vi "SimpleDemo - backup.vi"() -> ()   [LabVIEW 2011]
uses:
  C:/Users/Behavior Room/Desktop/Kinect Mouse/DepthSense/FunctionPointerProxy/FunctionPointerProxy/obj/Release/FunctionPointerProxy.dll
  FunctionPointerProxy/FunctionPointerProxy/obj/Release/FunctionPointerProxy.dll
  <userlib>/libOptrima-2-3/libOptrima-2-3.lvlib
  <vilib>/vision/Image Controls.llb/IMAQ Image.ctl
  Program Files (x86)/SoftKinetic/OptrimaSDK/lib/libOptrima-2-3.dll
  <vilib>/Platform/TimedLoop/XDataNode/XDataNode.xnode
  <vilib>/Platform/TimedLoop/XDataNode/nitl_modes.ctl
  <vilib>/Platform/TimedLoop/XDataNode/XDNodeRunTimeDep.lvlib
  <vilib>/Platform/TimedLoop/XDataNode/wakeup.ctl
  <vilib>/Platform/TimedLoop/XDataNode/timing_clust.ctl
panel:
  out "API version":string
  out "array length":i32
  out "Image":T1(plugin-control)
  out "add newframe\ncallback":i32
  in  "stop":bool
  in  "Buffer Size 3":i32=10
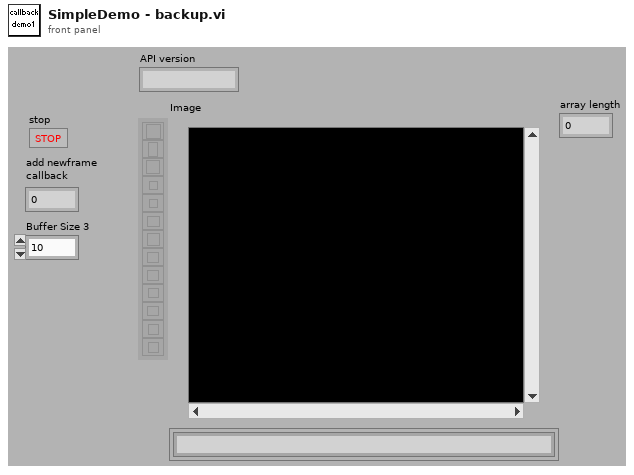
[diagram p1: front panel]
types:
  T1 = typedef "IMAQ Image.ctl" = refnum<image>
  T2 = typedef "XDNodeRunTimeDep.lvlib/timing_clust.ctl" = cluster{"Expected End [f-1]":u64, "Actual End [f-1]":u64, "Finished Late? [f-1]":bool, "Expected End [i-1]":u64, "Actual End [i-1]":u64, "Finished Late? [i-1]":bool, "Expected Start [i]":u64, "Actual Start [i]":u64, "Expected Start [f]":u64, "Actual Start [f]":u64, "Source Name":string, "Structure Name":string, "Period":i64, "Deadline":i64, "Offset":i64, "Start":i64, "Priority":i32, "Timeout":i32, "Mode":T3, "Wakeup Reason":T4, "Error":errorcluster, "Source Type":string, "Secondary Source Type":string, "Global End Time":u64, "Global Start Time":u64, "Frame Duration":u64, "Iteration Duration":u64, "Assigned CPU":i32, "I/O Scan Engine Mode":u32}
  T3 = typedef "XDNodeRunTimeDep.lvlib/nitl_modes.ctl" = enum32{"No Change", "Process missed periods, maintain original phase", "Discard missed periods, maintain original phase", "Process missed periods, ignore original phase", "Discard missed periods, ignore original phase"}
  T4 = typedef "XDNodeRunTimeDep.lvlib/wakeup.ctl" = enum32{"Normal", "Aborted", "Asynchronous wakeup", "Timing source error", "Timed loop error", "Timeout"}
  T5 = cluster{"queue out":refnum<queue>, "queue out":refnum<queue>}
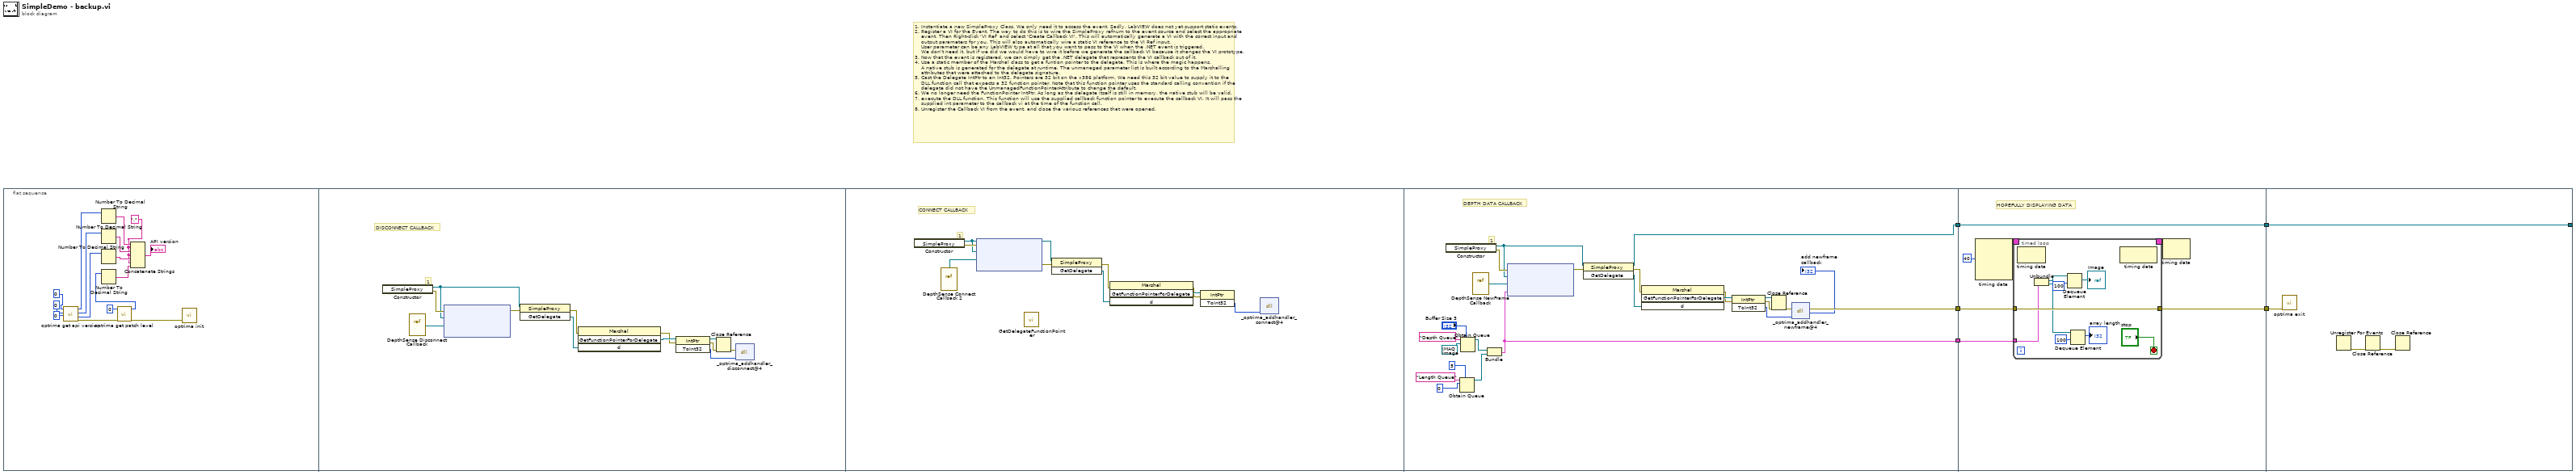
[diagram p0: block diagram]
diagram:
  # "1. Instantiate a new SimpleProxy Class. We only need it to access the event. Sadly, LabVIEW does not yet support static events.\n2. Register a VI for the Event. The way to do this is to wire the SimpleProxy refnum to the event source and select the appropriate\n    event. Then Right-click 'VI Ref' and select 'Create Callback VI'. This will automatically generate a VI with the correct input and\n    output parameters for you. This will also automatically wire a static VI reference to the VI Ref input.\n    User parameter can be any LabVIEW type at all that you want to pass to the VI when the .NET event is triggered.\n    We don't need it, but if we did we would have to wire it before we generate the callback VI because it changes the VI prototype.\n3. Now that the event is registered, we can simply get the .NET delegate that represents the VI callback out of it.\n4. Use a static member of the Marshal class to get a funtion pointer to the delegate. This is where the magic happens.\n    A native stub is generated for the delegate at runtime. The unmanaged parameter list is built according to the Marshalling\n    attributes that were attached to the delegate signature.\n5. Cast the Delegate IntPtr to an Int32. Pointers are 32 bit on the x386 platform. We need this 32 bit value to supply it to the\n    DLL function call that expects a 32 function pointer. Note that this function pointer uses the standard calling convention if the\n    delegate did not have the UnmanagedFunctionPointerAttribute to change the default.\n6. We no longer need the FunctionPointer IntPtr. As long as the delegate itself is still in memory, the native stub will be valid.\n7. execute the DLL function. This function will use the supplied callback function pointer to execute the callback VI. It will pass the\n    supplied int parameter to the callback vi at the time of the function call.\n8. Unregister the Callback VI from the event, and close the various references that were opened."
  n1 = flat-sequence {
    tunnel: [w66] -> w5
    tunnel: [w64] -> w4
    tunnel: [w44] -> w3
    tunnel: w5 -> [w73]
    tunnel: w4 -> [w71]
    tunnel: w3 -> [w70]
    tunnel: [w72] -> w2
    tunnel: [w71] -> w1
    tunnel: [w92] -> _
    tunnel: w2 -> [w91]
    tunnel: w1 -> [w92]
    frame #0 {
      w6 = "."
      n2 = call <userlib>:"optrima get api version.vi"("minor"=u32 0, "major"=u32 0, "release"=u32 0) -> ("error out"=w21:errorcluster, "minor out"=w17:u32, "major out"=w18:u32, "release out"=w19:u32)  [unwired: 5 in]
      n3 = Number To Decimal String(number=w19) -> (decimal integer string=w15:string)  [unwired: 1 in]
      n4 = Number To Decimal String(number=w18) -> (decimal integer string=w9:string)  [unwired: 1 in]
      n5 = Number To Decimal String(number=w17) -> (decimal integer string=w8:string)  [unwired: 1 in]
      n6 = call <userlib>:"optrima get patch level.vi"("error in (no error)"=w21, "patch"=u32 0) -> ("error out"=w20:errorcluster, "patch out"=w16:u32)  [unwired: 8 in]
      n7 = Number To Decimal String(number=w16) -> (decimal integer string=w7:string)  [unwired: 1 in]
      n8 = Concatenate Strings(w15, w6, w9, w6, w8, w6, w7) -> (→"API version":string)
      n9 = call <userlib>:"optrima init.vi"("error in (no error)"=w20) -> ()  [unwired: 10 in, 1 out]
    }
    frame #1 {
      # "DISCONNECT CALLBACK"
      # "1"
      n10 = constructor class="SimpleProxy"() -> (reference out=w25:refnum<k24>, error out=w29:errorcluster)  [unwired: 3 in, 1 out]
      n11 = vi-ref "DepthSense Disconnect Callback.vi"() -> ("vi reference"=w23:refnum<vi>)
      n12 = node(w29, w25, w23) -> (w33:errorcluster)  [unwired: 2 in, 1 out]
      n13 = invoke class="SimpleProxy" method="GetDelegate"(reference=w25, error in=w33) -> (error out=w31:errorcluster, "GetDelegate"=w22:refnum<k24>)  [unwired: 1 in, 1 out]
      n14 = invoke class="Marshal" method="GetFunctionPointerForDelegate"(error in=w31, "d"=w22) -> (error out=w30:errorcluster, "GetFunctionPointerForDelegate"=w32:refnum<k24>)  [unwired: 2 in, 2 out]
      n15 = invoke class="IntPtr" method="ToInt32"(reference=w32, error in=w30) -> (reference out=w28:refnum<k24>, error out=w26:errorcluster, "ToInt32"=w24:i32)  [unwired: 1 in]
      n16 = Close Reference(reference=w28, error in (no error)=w26) -> (error out=w27:errorcluster)
      n17 = dll-call lib="C:/Program Files (x86)/SoftKinetic/OptrimaSDK/lib/libOptrima-2-3.dll" fn="_optrima_addhandler_disconnect@4"(error in=w27, "handlerfunc"=w24) -> ()  [unwired: 4 in, 2 out]
    }
    frame #2 {
      # "CONNECT CALLBACK"
      # "1"
      n18 = constructor class="SimpleProxy"() -> (reference out=w37:refnum<k24>, error out=w38:errorcluster)  [unwired: 3 in, 1 out]
      n19 = vi-ref "DepthSense Connect Callback 2.vi"() -> ("vi reference"=w35:refnum<vi>)
      n20 = node(w38, w37, w35) -> (w42:errorcluster)  [unwired: 2 in, 1 out]
      n21 = call "GetDelegateFunctionPointer.vi"() -> ()  [unwired: 9 in, 3 out]
      n22 = invoke class="SimpleProxy" method="GetDelegate"(reference=w37, error in=w42) -> (error out=w40:errorcluster, "GetDelegate"=w34:refnum<k24>)  [unwired: 1 in, 1 out]
      n23 = invoke class="Marshal" method="GetFunctionPointerForDelegate"(error in=w40, "d"=w34) -> (error out=w39:errorcluster, "GetFunctionPointerForDelegate"=w41:refnum<k24>)  [unwired: 2 in, 2 out]
      n24 = invoke class="IntPtr" method="ToInt32"(reference=w41, error in=w39) -> ("ToInt32"=w36:i32)  [unwired: 1 in, 2 out]
      n25 = dll-call lib="C:/Program Files (x86)/SoftKinetic/OptrimaSDK/lib/libOptrima-2-3.dll" fn="_optrima_addhandler_connect@4"("handlerfunc"=w36) -> ()  [unwired: 5 in, 2 out]
    }
    frame #3 {
      # "DEPTH DATA CALLBACK"
      # "1"
      n26 = constructor class="SimpleProxy"() -> (reference out=w55:refnum<k24>, error out=w59:errorcluster)  [unwired: 3 in, 1 out]
      n27 = Obtain Queue(max queue size (-1, unlimited)=5, name (unnamed)="Length Queue", element data type=0) -> (queue out=w45:refnum<queue>)  [unwired: 2 in, 2 out]
      n28 = Obtain Queue(max queue size (-1, unlimited)="Buffer Size 3", name (unnamed)="Depth Queue", element data type=T1 refnum ("New Image")) -> (queue out=w49:refnum<queue>)  [unwired: 2 in, 2 out]
      n29 = vi-ref "DepthSense NewFrame Callback.vi"() -> ("vi reference"=w43:refnum<vi>)
      n30 = Bundle("queue out"=w49, "queue out"=w45) -> (w44:T5)  [unwired: 1 in]
      n31 = node(w59, w55, w43, w44) -> (w63:errorcluster)  [unwired: 1 in, 1 out]
      n32 = invoke class="SimpleProxy" method="GetDelegate"(reference=w55, error in=w63) -> (reference out=w64:refnum<k24>, error out=w61:errorcluster, "GetDelegate"=w65:refnum<k24>)  [unwired: 1 in]
      n33 = invoke class="Marshal" method="GetFunctionPointerForDelegate"(error in=w61, "d"=w65) -> (error out=w60:errorcluster, "GetFunctionPointerForDelegate"=w62:refnum<k24>)  [unwired: 2 in, 2 out]
      n34 = invoke class="IntPtr" method="ToInt32"(reference=w62, error in=w60) -> (reference out=w58:refnum<k24>, error out=w56:errorcluster, "ToInt32"=w54:i32)  [unwired: 1 in]
      n35 = Close Reference(reference=w58, error in (no error)=w56) -> (error out=w57:errorcluster)
      n36 = dll-call lib="C:/Program Files (x86)/SoftKinetic/OptrimaSDK/lib/libOptrima-2-3.dll" fn="_optrima_addhandler_newframe@4"(error in=w57, "handlerfunc"=w54) -> (error out=w66:errorcluster, "return type"=→"add newframe\ncallback":i32)  [unwired: 3 in, 1 out]
    }
    frame #4 {
      # "HOPEFULLY DISPLAYING DATA"
      n37 = node-c288(i64 40 ("Period")) -> (w69:T2)  [unwired: 3 in]
      n38 = timed-loop {
        tunnel: [w81] -> w72
        tunnel: w73 -> [w81]
        tunnel: w70 -> [w80]
        timing: w69 -> [_]
        timing-out: [_] -> w68
        stop <- "stop" stop-if-true
        n39 = node-c288() -> ()  [unwired: 1 in, 1 out]
        n40 = Unbundle(w80) -> ("queue out"=w78:refnum<queue>, "queue out"=w76:refnum<queue>)
        n41 = Dequeue Element(queue=w78, timeout in ms (-1)=100) -> (element=→"Image":T1)  [unwired: 1 in, 3 out]
        n42 = Dequeue Element(queue=w76, timeout in ms (-1)=100) -> (element=→"array length":i32)  [unwired: 1 in, 3 out]
        n43 = node-c288() -> ()  [unwired: 1 in, 1 out]
      }
      n44 = node-c288(w68) -> ()  [unwired: 1 out]
    }
    frame #5 {
      n45 = call <userlib>:"optrima exit.vi"("error in (no error)"=w91) -> ()  [unwired: 10 in, 1 out]
      n46 = Unregister For Events() -> (error out=w90:errorcluster)  [unwired: 2 in]
      n47 = Close Reference(error in (no error)=w90) -> (error out=w89:errorcluster)  [unwired: 1 in]
      n48 = Close Reference(error in (no error)=w89) -> ()  [unwired: 1 in, 1 out]
    }
  }
